vi "Destroy.vi"(0 "reference in":refnum<class "ZeroMQ.lvclass">, 5 "error in (no error)":errorcluster) -> (14 "reference out":refnum<class "ZeroMQ.lvclass">, 19 "error out":errorcluster)   [LabVIEW 2018, in "ZeroMQ.lvclass"]
uses:
  ZeroMQ.lvclass
  Communication_class/Communication.lvclass
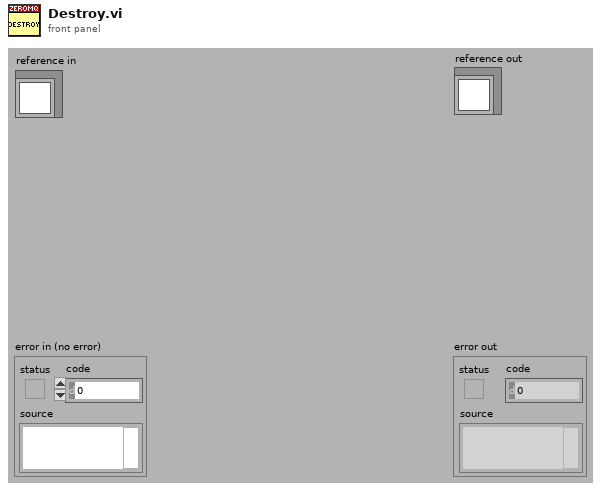
[diagram p1: front panel]
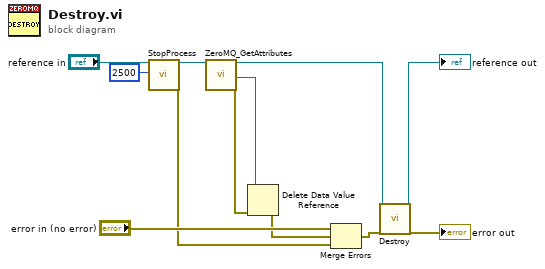
[diagram p0: block diagram]
diagram:
  n1 = call "StopProcess.vi"("reference in"="reference in", "ms timeout (-1)"=2500) -> ("reference out"=w3:refnum<class "ZeroMQ.lvclass">, "error out"=w1:errorcluster)  [unwired: 16 in]
  n2 = call "ZeroMQ_GetAttributes.vi"("reference in"=w3) -> ("reference out"=w8:refnum<class "ZeroMQ.lvclass">, "DataRef"=w11:refnum<data-value>, "error out"=w12:errorcluster)  [unwired: 15 in, 1 out]
  n3 = Delete Data Value Reference(data value reference=w11, error in=w12) -> (error out=w5:errorcluster)  [unwired: 1 out]
  n4 = Merge Errors("error in (no error)", w5, w1) -> (w10:errorcluster)
  n5 = call-parent "Destroy.vi"("reference in"=w8, "error in (no error)"=w10) -> ("reference out"=→"reference out":refnum<class "ZeroMQ.lvclass">, "error out"=→"error out":errorcluster)  [unwired: 16 in]
